vi "Read HTTP Session.vi"(8 "error in (no error)":errorcluster, 11 "HTTP Session in":refnum<class "Session.lvclass">) -> (0 "error out":errorcluster, 2 "Client Handle":T1, 3 "HTTP Session out":refnum<class "Session.lvclass">)   [LabVIEW 2015, in "NI_Azure_Core.lvlib" / "Session.lvclass"]
uses:
  Session.lvclass
  <vilib>/httpClient/ClientHandle.ctl
  Session.lvclass/Session.ctl
  <vilib>/httpClient/LabVIEWHTTPClient.lvlib
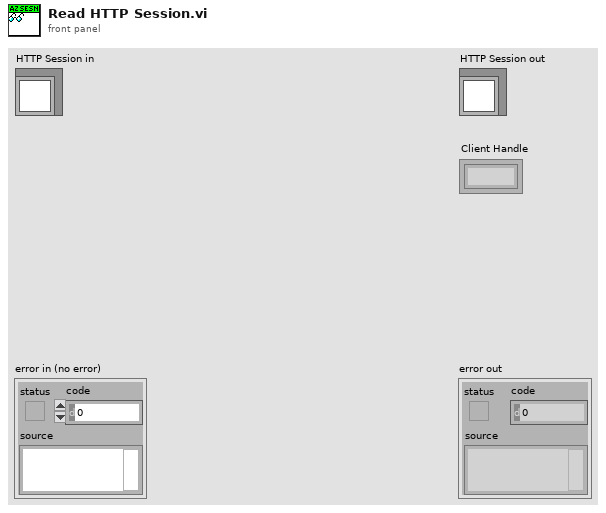
[diagram p1: front panel]
types:
  T1 = typedef "LabVIEWHTTPClient.lvlib/ClientHandle.ctl" = refnum<k1>
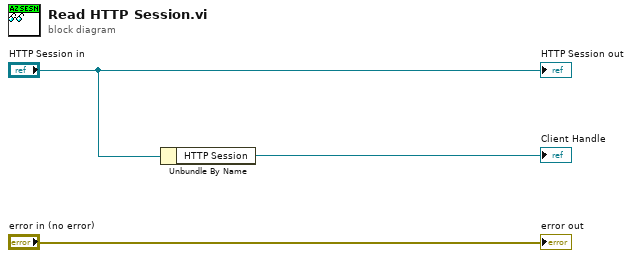
[diagram p0: block diagram]
diagram:
  n1 = Unbundle By Name("HTTP Session in") -> ("HTTP Session"=→"Client Handle":T1)
  "error out" <- "error in (no error)"
  "HTTP Session out" <- "HTTP Session in"
